vi "Update-buffer-contents.vi"(5 "UI buffer":refnum<notifier>, 6 "Frametime":dbl, 7 "Acq stats notif":refnum<notifier>, 8 "error in":errorcluster, 9 "Acquisition stats in":T1, 10 "Buffer element in":T2 {"Temperature characteristics"."Stand. dev. temperature" format="%#.1f"; "Temperature characteristics"."Min. temperature" format="%#.0f"; "Temperature characteristics"."Max. temperature" format="%#.0f"; "Temperature characteristics"."Average temperature" format="%#.0f"}, 11 "Buffers in":refnum<class "CV-Buffers.lvclass">) -> (0 "error IO":errorcluster, 1 "Acquisition stats":T1, 2 "Buffer element":T2 {"Temperature characteristics"."Stand. dev. temperature" format="%#.1f"; "Temperature characteristics"."Min. temperature" format="%#.0f"; "Temperature characteristics"."Max. temperature" format="%#.0f"; "Temperature characteristics"."Average temperature" format="%#.0f"}, 3 "Buffers":refnum<class "CV-Buffers.lvclass">, 4 "Data-loss?":bool)   [LabVIEW 2013, in "CameraVision.lvlib" / "CV-Main.lvclass"]
uses:
  CV-Main.lvclass
  Acquisition/Acquisition-stats.ctl
  Buffers/Storage-buffer.ctl
  <vilib>/vision/Image Controls.llb/IMAQ Image.ctl
  Temperature/Temperature-characteristics.ctl
  Analysis/Characteristics-cluster.ctl
  Buffers/CV-Buffers.lvclass
  Buffers/CV-Buffers.lvclass/CV-Buffers.ctl
  Buffers/Mapping-buffer.ctl
  Buffers/Read Storage buffer.vi
  Buffers/Read Mapping buffer.vi
  Temperature/CV-Temperature.lvclass
  Analysis/CV-Analysis.lvclass
  Acquisition/CV-Acquisition.lvclass
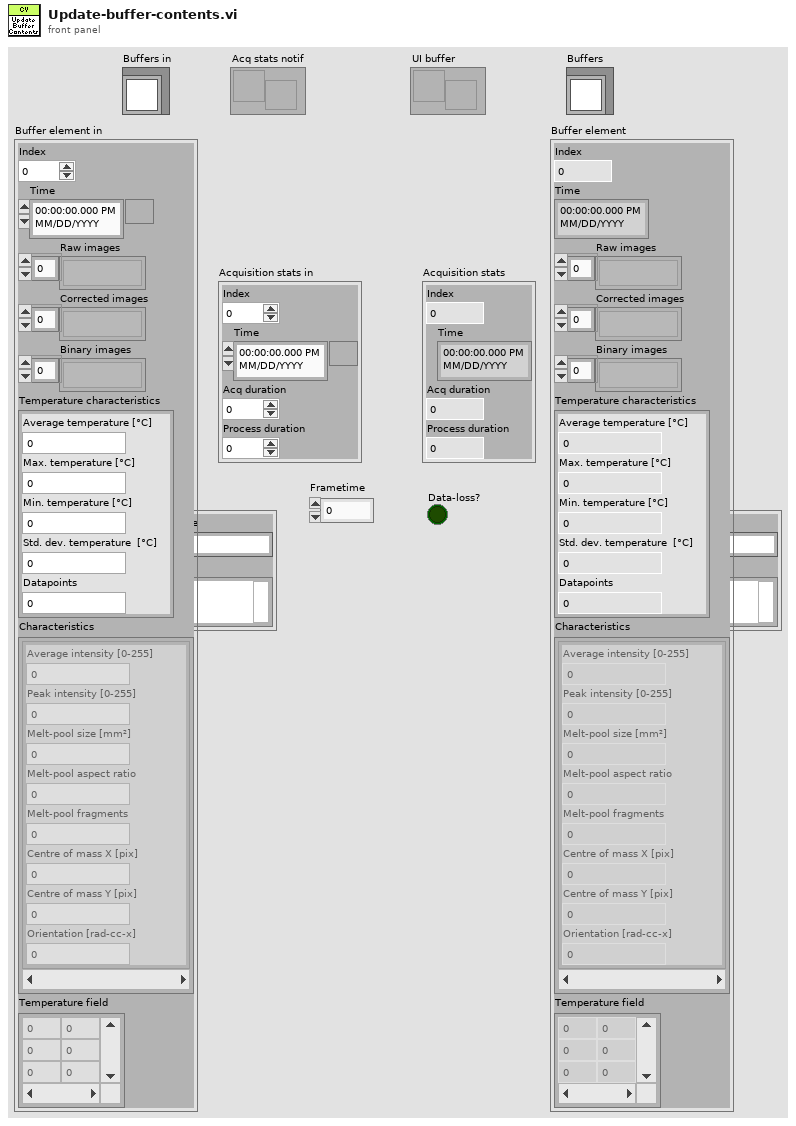
[diagram p1: front panel]
types:
  T1 = typedef "CameraVision.lvlib/CV-Acquisition.lvclass/Acquisition-stats.ctl" = cluster{"Index":i32, "Time":timestamp, "Acq duration":dbl, "Process duration":dbl}
  T2 = typedef "CameraVision.lvlib/CV-Buffers.lvclass/Storage-buffer.ctl" = cluster{"Index":i32, "Time":timestamp, "Raw images":T3[], "Corrected images":T3[], "Binary images":T3[], "Temperature characteristics":T4, "Characteristics":T5[], "Temperature field":dbl[][]}
  T3 = typedef "IMAQ Image.ctl" = refnum<image>
  T4 = typedef "CameraVision.lvlib/CV-Temperature.lvclass/Temperature-characteristics.ctl" = cluster{"Average temperature ":dbl, "Max. temperature":dbl, "Min. temperature":dbl, "Stand. dev. temperature":dbl, "Datapoints":dbl}
  T5 = typedef "CameraVision.lvlib/CV-Analysis.lvclass/Characteristics-cluster.ctl" = cluster{"Average intensity":dbl, "Peak intensity":dbl, "Melt-pool size":dbl, "Melt-pool aspect ratio":dbl, "Melt-pool fragments":dbl, "Centre of mass X":dbl, "Centre of mass Y":dbl, "Orientation":dbl}
  T6 = typedef "CameraVision.lvlib/CV-Buffers.lvclass/Mapping-buffer.ctl" = cluster{"Time":timestamp, "Index":i32, "Temperature characteristics":T4, "Characteristics":T5[], "Xcoord":sgl, "Ycoord":sgl}
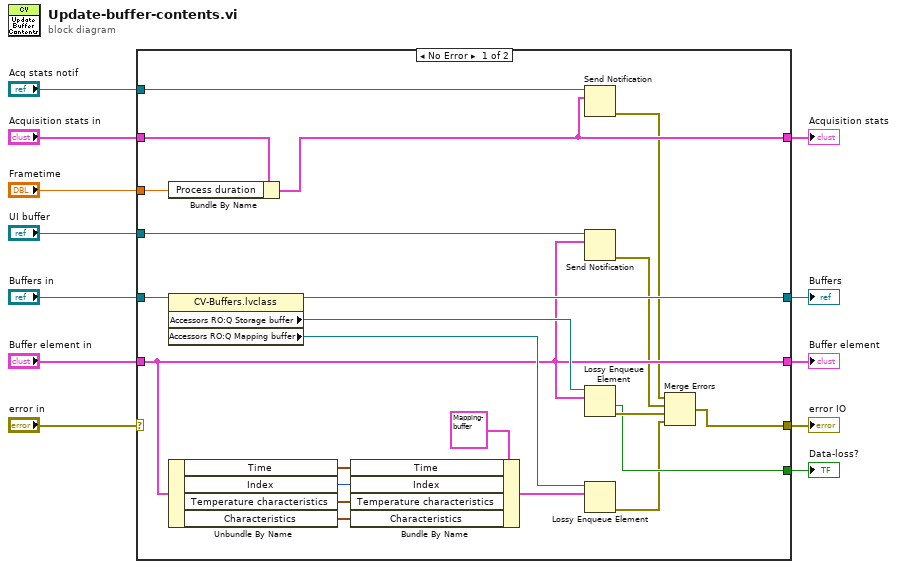
[diagram p0: block diagram]
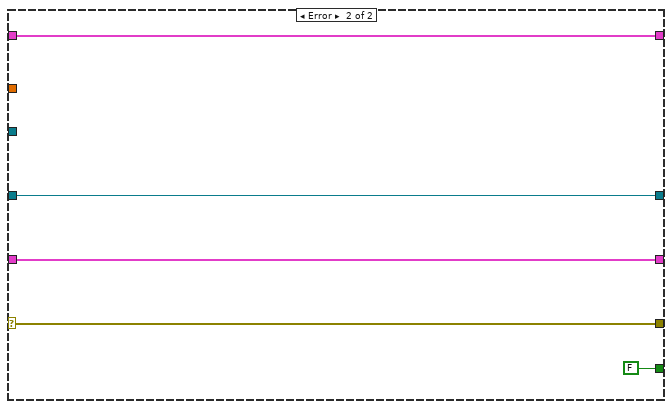
[diagram p2: hidden frame]
diagram:
  n1 = case shown="No Error" "error in" {
    selector: "error in" -> [_ w39]
    tunnel: [w27 w39] -> w11
    tunnel: "Frametime" -> [w34 _]
    tunnel: "Buffer element in" -> [w15 w38]
    tunnel: "Buffers in" -> [w32 w37]
    tunnel: "Acquisition stats in" -> [w33 w36]
    tunnel: "Acq stats notif" -> [w31 _]
    tunnel: [w29 w37] -> w4
    tunnel: [w15 w38] -> w5
    tunnel: [w22 w36] -> w3
    tunnel: [w26 FALSE ("overflow?")] -> w2
    tunnel: "UI buffer" -> [w16 _]
    frame No Error {
      n2 = Bundle By Name(cluster=w33, "Process duration"=w34) -> (w22:T1)
      n3 = property class="CV-Buffers.lvclass"(reference=w32) -> (reference out=w29:refnum<class "CV-Buffers.lvclass">, "Accessors RO:Q Storage buffer"=w30:refnum<queue>, "Accessors RO:Q Mapping buffer"=w24:refnum<queue>)  [unwired: 1 in, 1 out]
      n4 = Unbundle By Name(w15) -> ("Time"=w21:timestamp, "Index"=w20:i32, "Temperature characteristics"=w19:T4, "Characteristics"=w18:T5[])
      n5 = Bundle By Name(cluster=T6 {"Time"=timestamp(0 s since 1904-01-01), "Index"=0, "Temperature characteristics"={"Average temperature "=0.0, "Max. temperature"=0.0, "Min. temperature"=0.0, "Stand. dev. temperature"=0.0, "Datapoints"=0.0}, "Characteristics"=[], "Xcoord"=0.0, "Ycoord"=0.0} ("element"), "Time"=w21, "Index"=w20, "Temperature characteristics"=w19, "Characteristics"=w18) -> (w17:T6)
      n6 = Send Notification(notification=w22, notifier=w31) -> (error out=w14:errorcluster)  [unwired: 1 in, 1 out]
      n7 = Send Notification(notification=w15, notifier=w16) -> (error out=w13:errorcluster)  [unwired: 1 in, 1 out]
      n8 = Lossy Enqueue Element(queue=w30, element=w15) -> (overflow?=w26:bool, error out=w28:errorcluster)  [unwired: 1 in, 2 out]
      n9 = Lossy Enqueue Element(queue=w24, element=w17) -> (error out=w25:errorcluster)  [unwired: 1 in, 3 out]
      n10 = Merge Errors(w14, w13, w28, w25) -> (w27:errorcluster)
    }
    frame Error {
    }
  }
  "error IO" <- w11
  "Buffer element" <- w5
  "Buffers" <- w4
  "Acquisition stats" <- w3
  "Data-loss?" <- w2
